vi "Parse Subcommand.vi"(0 "Text In":string, 7 "Subcommands":string[](array[string]), 9 "Parameters":i32[](array[numeric])) -> (3 "Done":bool, 4 "Text Out":string, 8 "Subcommand":string, 10 "# of Parameters":i32, 12 "Parameter 3":string, 13 "Parameter 2":string, 14 "Parameter 1":string)   [LabVIEW 2015]
doc: "Parses the subcommands from a line."
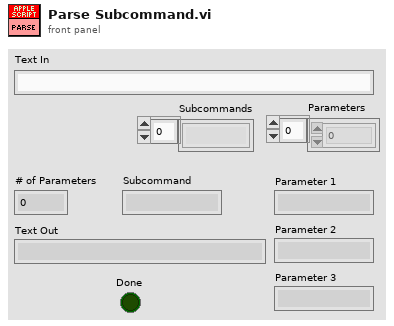
[diagram p1: front panel]
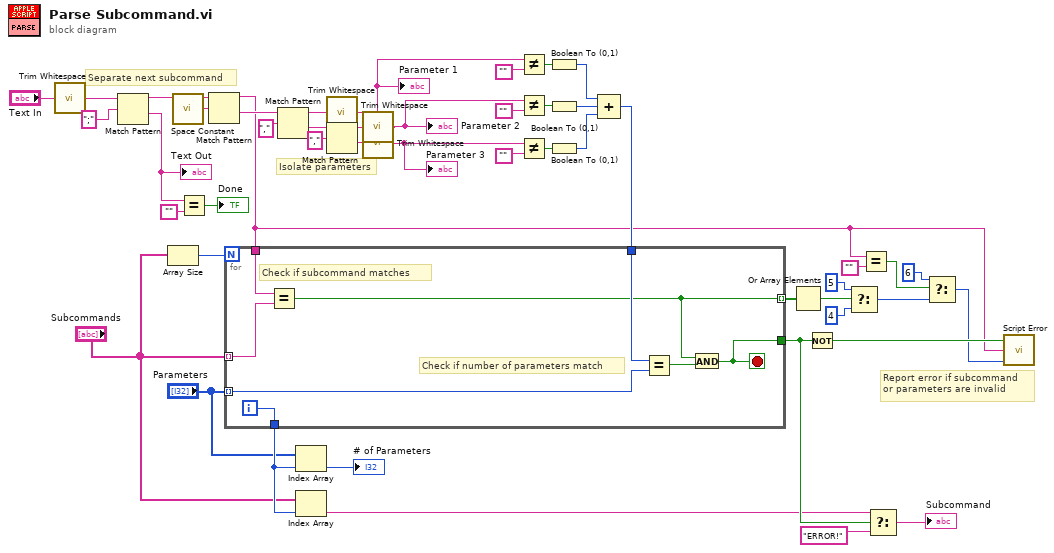
[diagram p0: block diagram]
diagram:
  # "Report error if subcommand\nor parameters are invalid"
  # "Separate next subcommand"
  # "Isolate parameters"
  n1 = call <vilib>:"Trim Whitespace.vi"("string"="Text In") -> ("trimmed string"=w14:string)  [unwired: 1 in]
  n2 = Match Pattern(string=w14, regular expression=";") -> (before substring=w10:string, after substring=w8:string)  [unwired: 1 in, 2 out]
  "Text Out" <- w8
  n3 = Array Size(array="Subcommands") -> (size(s)=w42:i32)
  n4 = call <vilib>:"Space Constant.vi"() -> ("String"=w12:string)
  n5 = Equal?(x=w8, y="") -> (x = y?=→"Done":bool)
  n6 = Match Pattern(string=w10, regular expression=w12) -> (before substring=w5:string, after substring=w9:string)  [unwired: 1 in, 2 out]
  n7 = Match Pattern(string=w9, regular expression=",") -> (before substring=w17:string, after substring=w41:string)  [unwired: 1 in, 2 out]
  n8 = call <vilib>:"Trim Whitespace.vi"("string"=w17) -> ("trimmed string"=w16:string)  [unwired: 1 in]
  "Parameter 1" <- w16
  n9 = Match Pattern(string=w41, regular expression=",") -> (before substring=w21:string, after substring=w19:string)  [unwired: 1 in, 2 out]
  n10 = call <vilib>:"Trim Whitespace.vi"("string"=w21) -> ("trimmed string"=w20:string)  [unwired: 1 in]
  "Parameter 2" <- w20
  n11 = call <vilib>:"Trim Whitespace.vi"("string"=w19) -> ("trimmed string"=w18:string)  [unwired: 1 in]
  "Parameter 3" <- w18
  n12 = Not Equal?(x=w16, y="") -> (x != y?=w33:bool)
  n13 = Not Equal?(x=w20, y="") -> (x != y?=w34:bool)
  n14 = Not Equal?(x=w18, y="") -> (x != y?=w35:bool)
  n15 = Boolean To (0,1)(Boolean=w33) -> (0, 1=w36:i16)
  n16 = Boolean To (0,1)(Boolean=w34) -> (0, 1=w37:i16)
  n17 = Boolean To (0,1)(Boolean=w35) -> (0, 1=w38:i16)
  n18 = Compound Arithmetic op=ADD(w36, w37, w38) -> (w22:i16)
  n19 = for {
    N: w42 -> [_]
    tunnel: "Subcommands" -> [w55] mode=indexing
    tunnel: "Parameters" -> [w54] mode=indexing
    tunnel: [w53] -> w48
    tunnel: [w52] -> w27
    tunnel: w22 -> [w51]
    tunnel: w5 -> [w50]
    tunnel: [w49] -> w29 mode=indexing
    i -> [w53]
    stop <- w52 stop-if-true
    # "Check if number of parameters match"
    # "Check if subcommand matches"
    n20 = Equal?(x=w50, y=w55) -> (x = y?=w49:bool)
    n21 = Equal?(x=w51, y=w54) -> (x = y?=w56:bool)
    n22 = And(x=w49, y=w56) -> (x .and. y?=w52:bool)
  }
  n23 = Index Array(array="Parameters", index=w48) -> (element=→"# of Parameters":i32)
  n24 = Index Array(array="Subcommands", index=w48) -> (element=w26:string)
  n25 = Or Array Elements(Boolean array=w29) -> (logical OR=w25:bool)
  n26 = Not(x=w27) -> (.not. x?=w6:bool)
  n27 = Select(t=5 ("Error Code"), s=w25, f=4 ("Error Code")) -> (s? t:f=w3:i32)
  n28 = Equal?(x=w5, y="") -> (x = y?=w2:bool)
  n29 = Select(t=w26, s=w27, f="ERROR!") -> (s? t:f=→"Subcommand":string)
  n30 = Select(t=6 ("Error Code"), s=w2, f=w3) -> (s? t:f=w1:i32)
  n31 = call "Script Error.vi"("Error?"=w6, "Error Details"=w5, "Error Code"=w1) -> ()  [unwired: 2 in, 1 out]
